vi "DBL U64 Binary View.vi"() -> ()   [LabVIEW 2016]
panel:
  out "DBL":dbl
  out "U64 as U8s reversed 1":u8[](array[numeric]) format="%08b"
  out "DBL as U8s 1":u8[](array[numeric]) format="%08b"
  out "U64 as U8s 1":u8[](array[numeric]) format="%08b"
  out "U64 Binary 1":u64 format="%064b"
  out "DBL Binary 1":u64 format="%064b"
  in  "U64 1":u64=14200896
  in  "DBL 1":dbl=4312.0
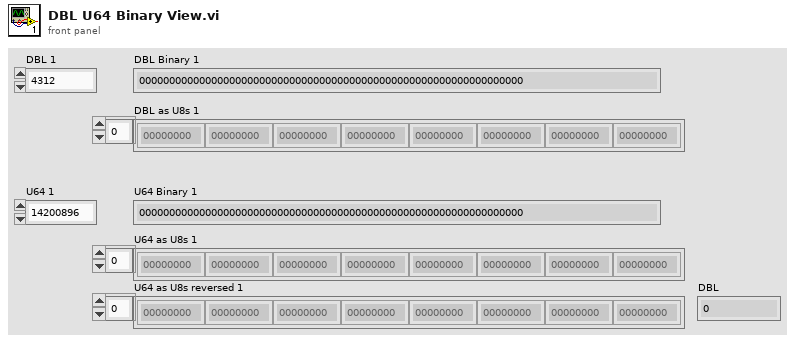
[diagram p1: front panel]
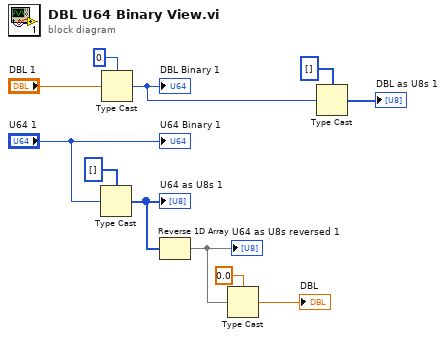
[diagram p0: block diagram]
diagram:
  n1 = Type Cast(type=u8[] [], x="U64 1") -> (*(type *) &x=w4:u8[])
  "U64 as U8s 1" <- w4
  n2 = Type Cast(type=u64 0, x="DBL 1") -> (*(type *) &x=w5:u64)
  "DBL Binary 1" <- w5
  n3 = Reverse 1D Array(array=w4) -> (reversed array=w3:u8[])
  "U64 as U8s reversed 1" <- w3
  n4 = Type Cast(type=0.0, x=w3) -> (*(type *) &x=→"DBL":dbl)
  n5 = Type Cast(type=u8[] [], x=w5) -> (*(type *) &x=→"DBL as U8s 1":u8[])
  "U64 Binary 1" <- "U64 1"
